vi "Main.vi"() -> ()   [LabVIEW 2017, in "Composite Pattern Demo.lvclass"]
uses:
  Composite Pattern Demo.lvclass
  Composite Employee Class/Composite Employee.lvclass
panel:
  out "Employee List":string[](array[string])
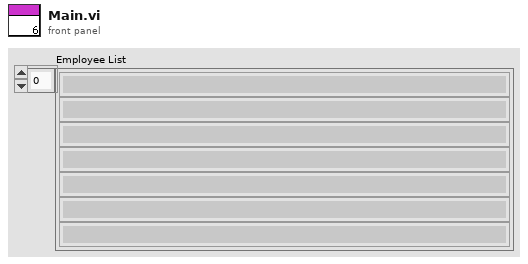
[diagram p1: front panel]
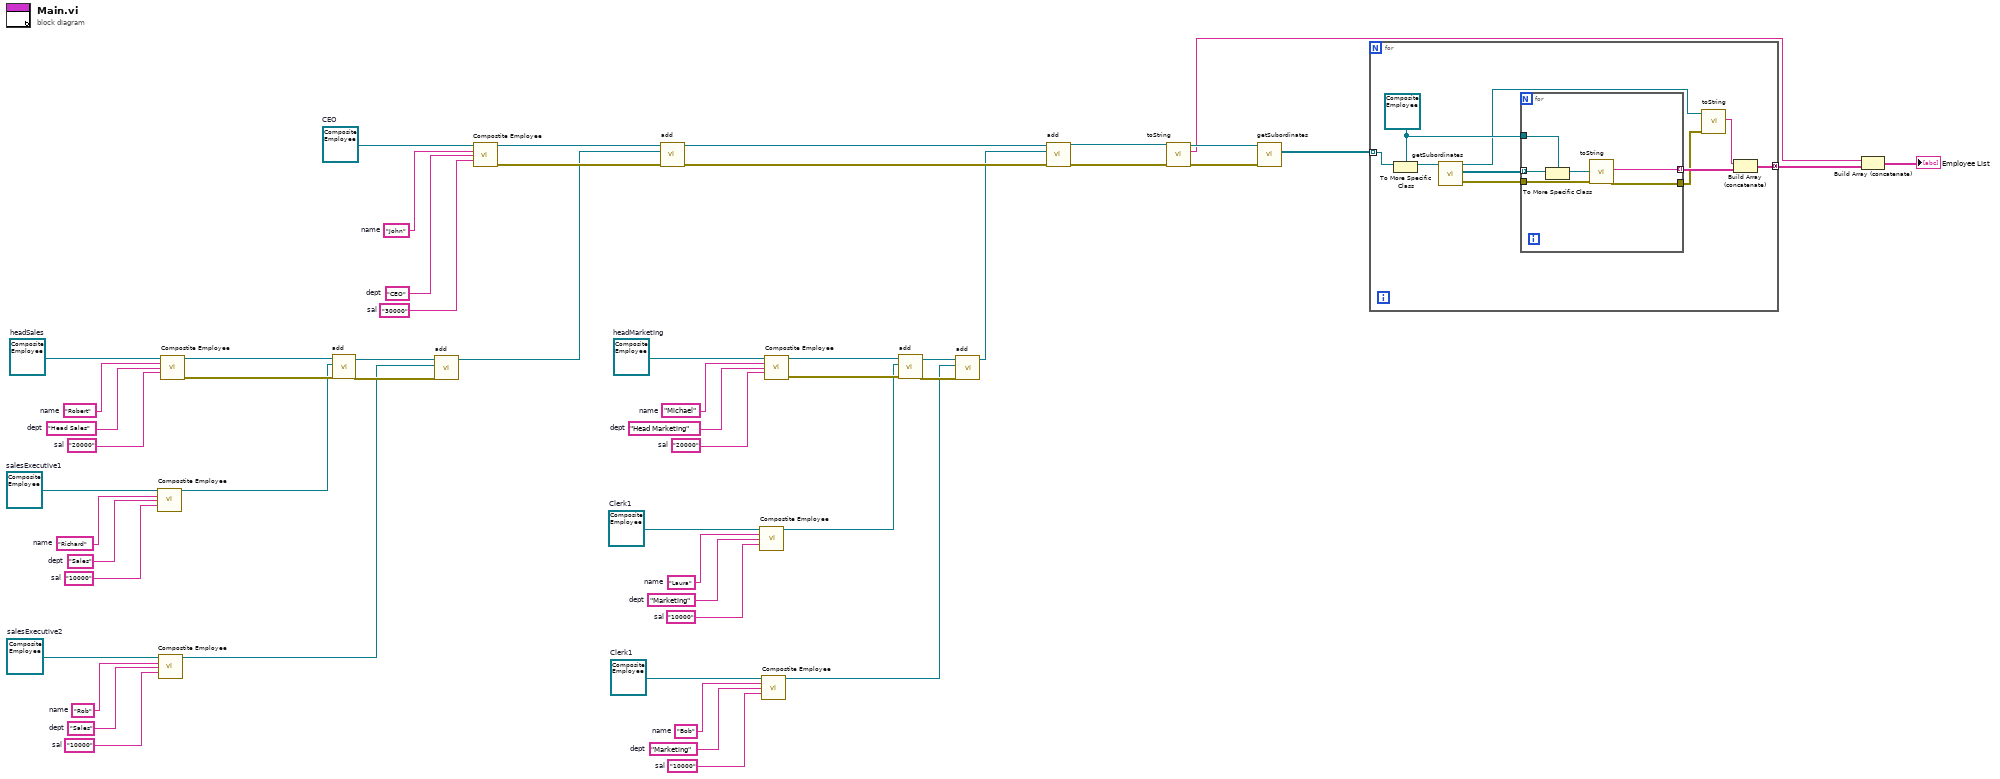
[diagram p0: block diagram]
diagram:
  w27 = "10000"  # sal
  w28 = "Sales"  # dept
  w29 = "Rob"  # name
  w30 = refnum<class "Composite Employee.lvclass"> refnum  # salesExecutive2
  w34 = "10000"  # sal
  w33 = "Sales"  # dept
  w32 = "Richard"  # name
  w31 = refnum<class "Composite Employee.lvclass"> refnum  # salesExecutive1
  w35 = "10000"  # sal
  w36 = "Marketing"  # dept
  w37 = "Bob"  # name
  w38 = refnum<class "Composite Employee.lvclass"> refnum  # Clerk1
  w42 = "10000"  # sal
  w41 = "Marketing"  # dept
  w40 = "Laura"  # name
  w39 = refnum<class "Composite Employee.lvclass"> refnum  # Clerk1
  w43 = "20000"  # sal
  w44 = "Head Marketing"  # dept
  w45 = "Michael"  # name
  w46 = refnum<class "Composite Employee.lvclass"> refnum  # headMarketing
  w50 = "20000"  # sal
  w49 = "Head Sales"  # dept
  w48 = "Robert"  # name
  w47 = refnum<class "Composite Employee.lvclass"> refnum  # headSales
  w51 = "30000"  # sal
  w52 = "CEO"  # dept
  w53 = "John"  # name
  w54 = refnum<class "Composite Employee.lvclass"> refnum  # CEO
  n1 = call-dynamic "Compostite Employee.vi"("Composite Employee in"=w31, "name"=w32, "dept"=w33, "sal"=w34) -> ("Composite Employee out"=w18:refnum<class "Composite Employee.lvclass">)  [unwired: 10 in, 1 out]
  n2 = call-dynamic "Compostite Employee.vi"("Composite Employee in"=w30, "name"=w29, "dept"=w28, "sal"=w27) -> ("Composite Employee out"=w17:refnum<class "Composite Employee.lvclass">)  [unwired: 10 in, 1 out]
  n3 = call-dynamic "Compostite Employee.vi"("Composite Employee in"=w47, "name"=w48, "dept"=w49, "sal"=w50) -> ("Composite Employee out"=w20:refnum<class "Composite Employee.lvclass">, "error out"=w19:errorcluster)  [unwired: 10 in]
  n4 = call-dynamic "add.vi"("error in (no error)"=w19, "Composite Employee.lvclass"=w18, "Composite Employee in"=w20) -> ("error out"=w21:errorcluster, "Composite Employee out"=w22:refnum<class "Composite Employee.lvclass">)  [unwired: 7 in]
  n5 = call-dynamic "add.vi"("error in (no error)"=w21, "Composite Employee.lvclass"=w17, "Composite Employee in"=w22) -> ("Composite Employee out"=w16:refnum<class "Composite Employee.lvclass">)  [unwired: 7 in, 1 out]
  n6 = call-dynamic "Compostite Employee.vi"("Composite Employee in"=w54, "name"=w53, "dept"=w52, "sal"=w51) -> ("Composite Employee out"=w24:refnum<class "Composite Employee.lvclass">, "error out"=w23:errorcluster)  [unwired: 10 in]
  n7 = call-dynamic "add.vi"("error in (no error)"=w23, "Composite Employee.lvclass"=w16, "Composite Employee in"=w24) -> ("error out"=w25:errorcluster, "Composite Employee out"=w26:refnum<class "Composite Employee.lvclass">)  [unwired: 7 in]
  n8 = call-dynamic "Compostite Employee.vi"("Composite Employee in"=w39, "name"=w40, "dept"=w41, "sal"=w42) -> ("Composite Employee out"=w11:refnum<class "Composite Employee.lvclass">)  [unwired: 10 in, 1 out]
  n9 = call-dynamic "Compostite Employee.vi"("Composite Employee in"=w38, "name"=w37, "dept"=w36, "sal"=w35) -> ("Composite Employee out"=w10:refnum<class "Composite Employee.lvclass">)  [unwired: 10 in, 1 out]
  n10 = call-dynamic "Compostite Employee.vi"("Composite Employee in"=w46, "name"=w45, "dept"=w44, "sal"=w43) -> ("Composite Employee out"=w15:refnum<class "Composite Employee.lvclass">, "error out"=w14:errorcluster)  [unwired: 10 in]
  n11 = call-dynamic "add.vi"("error in (no error)"=w14, "Composite Employee.lvclass"=w11, "Composite Employee in"=w15) -> ("error out"=w12:errorcluster, "Composite Employee out"=w13:refnum<class "Composite Employee.lvclass">)  [unwired: 7 in]
  n12 = call-dynamic "add.vi"("error in (no error)"=w12, "Composite Employee.lvclass"=w10, "Composite Employee in"=w13) -> ("Composite Employee out"=w9:refnum<class "Composite Employee.lvclass">)  [unwired: 7 in, 1 out]
  n13 = call-dynamic "add.vi"("error in (no error)"=w25, "Composite Employee.lvclass"=w9, "Composite Employee in"=w26) -> ("error out"=w7:errorcluster, "Composite Employee out"=w8:refnum<class "Composite Employee.lvclass">)  [unwired: 7 in]
  n14 = call-dynamic "toString.vi"("error in (no error)"=w7, "Composite Employee in"=w8) -> ("error out"=w5:errorcluster, "resulting string"=w3:string, "Composite Employee out"=w6:refnum<class "Composite Employee.lvclass">)  [unwired: 7 in]
  n15 = call-dynamic "getSubordinates.vi"("error in (no error)"=w5, "Composite Employee in"=w6) -> ("subordinates"=w4:refnum<class "Employee.lvclass">[])  [unwired: 7 in, 2 out]
  n16 = for {
    tunnel: w4 -> [w64] mode=indexing
    tunnel: [w60] -> w1 mode=concatenating
    w56 = refnum<class "Composite Employee.lvclass"> refnum ("Composite Employee.lvclass")
    n17 = To More Specific Class(target class=w56, reference=w64) -> (specific class reference=w63:refnum<class "Composite Employee.lvclass">)  [unwired: 1 in, 1 out]
    n18 = call-dynamic "getSubordinates.vi"("Composite Employee in"=w63) -> ("error out"=w58:errorcluster, "subordinates"=w62:refnum<class "Employee.lvclass">[], "Composite Employee out"=w55:refnum<class "Composite Employee.lvclass">)  [unwired: 8 in]
    n19 = for {
      tunnel: w62 -> [w70] mode=indexing
      tunnel: [w68] -> w61 mode=indexing
      tunnel: w58 -> [w67]
      tunnel: [w66] -> w57
      tunnel: w56 -> [w65]
      n20 = To More Specific Class(target class=w65, reference=w70) -> (specific class reference=w69:refnum<class "Composite Employee.lvclass">)  [unwired: 1 in, 1 out]
      n21 = call-dynamic "toString.vi"("error in (no error)"=w67, "Composite Employee in"=w69) -> ("error out"=w66:errorcluster, "resulting string"=w68:string)  [unwired: 7 in, 1 out]
    }
    n22 = call-dynamic "toString.vi"("error in (no error)"=w57, "Composite Employee in"=w55) -> ("resulting string"=w59:string)  [unwired: 7 in, 2 out]
    n23 = Build Array (concatenate)(w59, w61) -> (w60:string[])
  }
  n24 = Build Array (concatenate)(w3, w1) -> (→"Employee List":string[])
